vi "OAT Analog Tacho Process (1 Tacho).vi"(0 "analog tacho signal":waveform(dbl)={"t0"=timestamp(0 s since 1904-01-01), "dt"=0.0, "Y"=[]}, 1 "missing pulses? (no:F)":bool, 2 "reset? (F)":bool, 5 "threshold (auto)":dbl=inf format="%.2f", 7 "pulse/revolution (1)":i32=1, 9 "hysteresis (0)":dbl format="%.2f", 11 "error in (no error)":errorcluster, 12 "pulse width (2)":i32=2, 13 "slope (Rising)":u16(ring) items=["Rising", "Falling"]) -> (4 "speed profile":T2 {"speed [RPM]" format="%.2f"; "time [s]" format="%.2f"}, 6 "actual threshold":dbl, 8 "speed position info":T1, 10 "no tacho?":bool, 15 "error out":errorcluster)   [LabVIEW 2017, in "SoundVib_TachProcess.lvlib"]
doc: "Locates tachometer pulse positions in analog tachometer signals using the number of generated pulses per revolution, the pulse width, and the arrival edge of the tachometer pulse. This VI also calculates the rotational speed of the device. Wire data to the <B>analog tacho signal</B> input to determine the polymorphic instance to use or manually select the instance."
uses:
  <vilib>/addons/Sound and Vibration/Order Analysis/Tach Process/SoundVib_TachProcess.lvlib
  <vilib>/addons/Sound and Vibration/Order Analysis/Tach Process/SubVIs/speed profile.ctl
  <vilib>/addons/Sound and Vibration/Order Analysis/Misc/OAT Position Info.ctl
  <vilib>/addons/_NISVFA/_Shared subVIs/Common/svc_Check for Waveform Parameter Continuity (no state).vi
  <vilib>/addons/_NISVFA/_Shared subVIs/Common/svc_Get SV Channel Info.vi
  <vilib>/addons/Sound and Vibration/Order Analysis/Tach Process/SubVIs/oa_Get Angular Speed (1 Tach).vi
  <vilib>/addons/Sound and Vibration/Order Analysis/Tach Process/SubVIs/OAT Edge Detection (1 Tach).vi
  <vilib>/Waveform/WDTOps.llb/WDT Waveform Duration DBL.vi
  <vilib>/addons/_NISVFA/_Shared subVIs/Common/svc_Engineering Units to Unit Label.vi
  <vilib>/addons/_NISVFA/_Shared subVIs/Common/svc_Unit Label to Engineering Units.vi
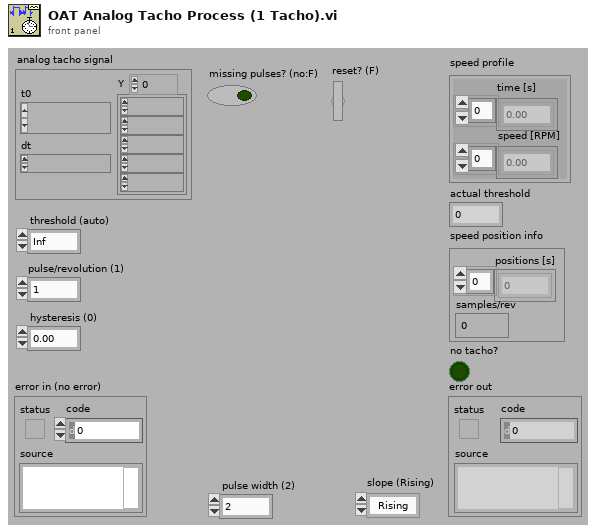
[diagram p1: front panel]
types:
  T1 = typedef "OAT Position Info.ctl" = cluster{"positions [s]":dbl[], "samples/rev":dbl}
  T2 = typedef "SoundVib_TachProcess.lvlib/speed profile.ctl" = cluster{"time [s]":dbl[], "speed [RPM]":dbl[]}
  T3 = cluster{"dt":bool, "t0 continuity":bool, "array length":bool, "channel info":bool, "name":bool}
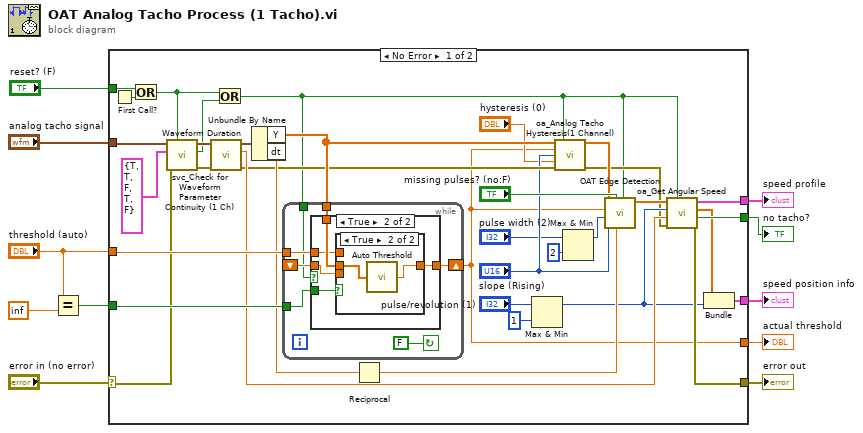
[diagram p0: block diagram]
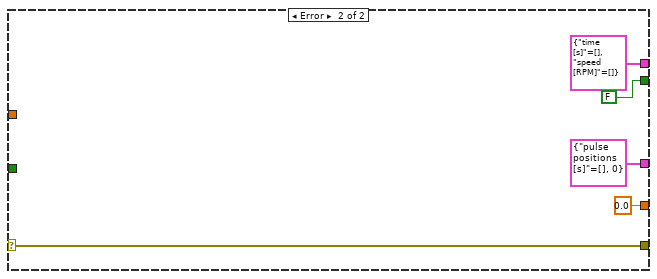
[diagram p4: hidden frame]
diagram:
  n1 = Equal?(x="threshold (auto)", y=inf) -> (x = y?=w7:bool)
  n2 = case shown="No Error" "error in (no error)" {
    selector: "error in (no error)" -> [w18 w68]
    tunnel: "analog tacho signal" -> [w21 _]
    tunnel: [w47 T2 {"time [s]"=[], "speed [RPM]"=[]} ("speed profile")] -> w10
    tunnel: [w43 w68] -> w9
    tunnel: w7 -> [w46 _]
    tunnel: "threshold (auto)" -> [w45 _]
    tunnel: [w44 FALSE ("No Tach? (False)")] -> w5
    tunnel: [w32 cluster{"pulse positions [s]":dbl[], i32} {"pulse positions [s]"=[], 0}] -> w3
    tunnel: "reset? (F)" -> [w13 _]
    tunnel: [w12 0.0 ("threshold")] -> w1
    frame No Error {
      n3 = First Call?() -> (First Call?: T/F=w31:bool)
      n4 = Or(x=w13, y=w31) -> (x .or. y?=w16:bool)
      n5 = call <vilib>:"svc_Check for Waveform Parameter Continuity (1 Ch).vi"("restart averaging (F)"=w16, "error in (no error)"=w18, "checks for channel parameter change"=T3 {"dt"=TRUE, "t0 continuity"=TRUE, "array length"=FALSE, "channel info"=TRUE, "name"=FALSE}, "scaled signal [EU]"=w21) -> ("error out"=w17:errorcluster, "waveform parameter changed"=w15:bool, "dup scaled signal [EU]"=w20:waveform(dbl))  [unwired: 2 in, 3 out]
      n6 = call-poly <vilib>:"Waveform Duration.vi"("error in (no error)"=w17, "waveform in"=w20) -> ("error out"=w28:errorcluster, "duration"=w36:dbl, "waveform out"=w35:waveform(dbl))  [unwired: 7 in]
      n7 = Or(x=w16, y=w15) -> (x .or. y?=w14:bool)
      n8 = Unbundle By Name(w35) -> ("Y"=w29:dbl[], "dt"=w41:dbl)
      n9 = while {
        tunnel: w29 -> [w54]
        shift-right: [w53] -> w12
        shift-left: _ -> [w52]
        tunnel: w14 -> [w49]
        tunnel: w46 -> [w48]
        tunnel: w45 -> [w50]
        stop <- FALSE continue-if-true
        n10 = case shown="True" w49 {
          tunnel: w54 -> [_ w60]
          tunnel: [w55 w59] -> w53
          tunnel: w52 -> [w55 w58]
          tunnel: w50 -> [_ w57]
          tunnel: w48 -> [_ w56]
          frame False {
          }
          frame True {
            n11 = case shown="True" w56 {
              tunnel: w60 -> [_ w63]
              tunnel: [w61 w62] -> w59
              tunnel: w58 -> [_ _]
              tunnel: w57 -> [w61 _]
              frame False {
              }
              frame True {
                n12 = call <vilib>:"Auto Threshold.vi"("x[n]"=w63) -> ("threshold"=w62:dbl)
              }
            }
          }
        }
      }
      n13 = Reciprocal(x=w41) -> (1/x=w40:dbl)
      n14 = Max & Min(x="pulse/revolution (1)", y=1) -> (max(x,y)=w33:i32)  [unwired: 1 out]
      n15 = call <vilib>:"oa_Analog Tacho Hysteresis(1 Channel).vi"("input signal"=w29, "reset? (T)"=w14, "threshold (auto)"=w12, "slope (Rising)"="slope (Rising)", "hysteresis(0)"="hysteresis (0)", "error in (no error)"=w28) -> ("output signal"=w30:dbl[], "error out"=w26:errorcluster)  [unwired: 8 in]
      n16 = Max & Min(x="pulse width (2)", y=2) -> (max(x,y)=w24:i32)  [unwired: 1 out]
      n17 = call-poly <vilib>:"OAT Edge Detection.vi"("reset? (True)"=w14, "sampling frequency [Hz]"=w40, "missing pulses? (no:F)"="missing pulses? (no:F)", "slope (Rising)"="slope (Rising)", "pulse width (2)"=w24, "threshold (0.0)"=w12, "x[n]"=w30) -> ("pulse positions [s]"=w37:dbl[])  [unwired: 3 in, 1 out]
      n18 = call-poly <vilib>:"oa_Get Angular Speed.vi"("reset? (True)"=w14, "error in (no error)"=w26, "input data duration [s]"=w36, "pulse/revolution (1)"=w33, "pulse positions [s]"=w37) -> ("error out"=w43:errorcluster, "no tacho? (F)"=w44:bool, "pulse positions [s]"=w34:dbl[], "speed profile"=w47:T2)  [unwired: 3 in]
      n19 = Bundle("pulse positions [s]"=w34, w33) -> (w32:cluster{"pulse positions [s]":dbl[], i32})  [unwired: 1 in]
    }
    frame Error {
    }
  }
  "speed profile" <- w10
  "speed position info" <- w3
  "error out" <- w9
  "no tacho?" <- w5
  "actual threshold" <- w1
